vi "NIST File Header.vi"(0 "reference in":refnum<class "WaveFile.lvclass">, 5 "error in (no error)":errorcluster, 7 "Wave File Path - READ":path) -> (14 "reference out":refnum<class "WaveFile.lvclass">, 19 "error out":errorcluster)   [LabVIEW 2020, in "WaveFile.lvclass"]
uses:
  WaveFile.lvclass
panel:
  out "Header":string[](array[string])
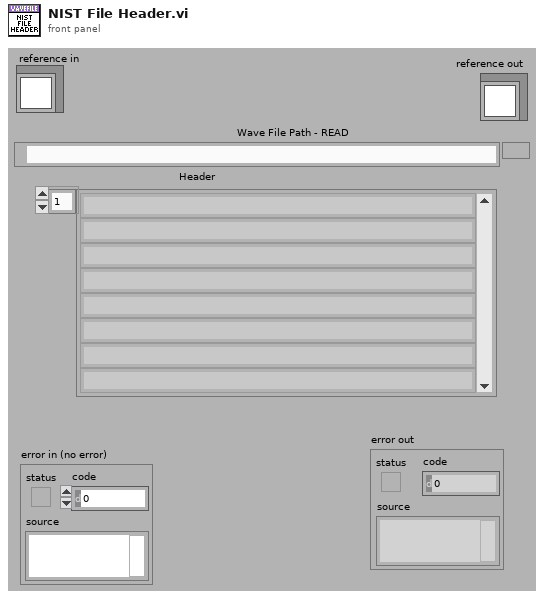
[diagram p1: front panel]
types:
  T1 = enum16{"big-endian, network order", "native, host order", "little-endian"}
  T2 = typedef "WaveFile.lvclass/ObjectAttributesRef.ctl" = refnum<data-value>
  T3 = typedef "WaveFile.lvclass/ObjectAttributes.ctl" = cluster{"Time Data":refnum<class "GSwFormDSP.lvclass">, "New Time Data Obj?":bool, "NIST File Header":T4}
  T4 = typedef "WaveFile.lvclass/NIST File Header.ctl" = cluster{"Version":string, "Header Nb Bytes":i32, "Nb Samples":i32, "Nb Bytes/sample":i32, "Nb Channels":i32, "byte order":enum16{"big-endian, network order", "native, host order", "little-endian"}, "Fs":dbl, "Valid Header?":bool}
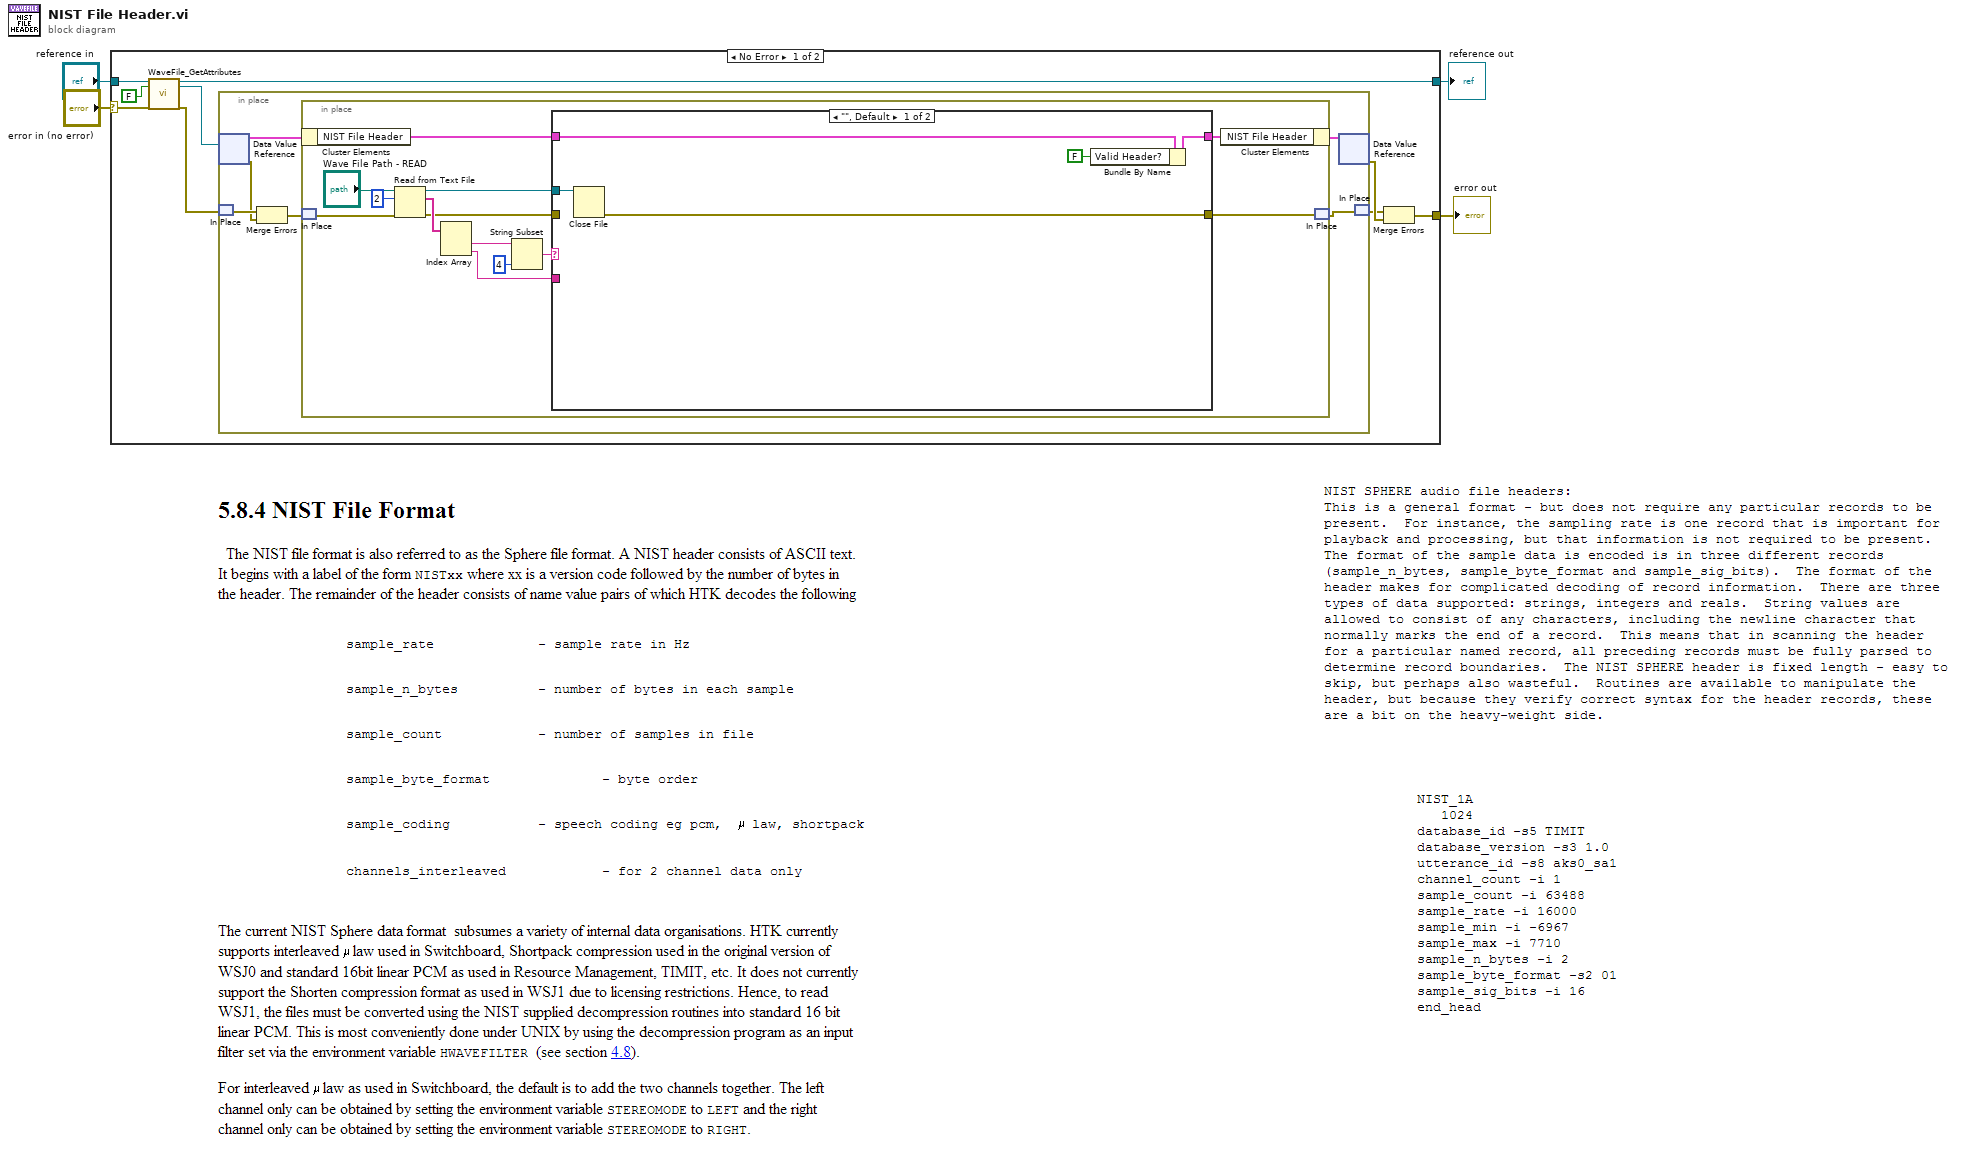
[diagram p0: block diagram]
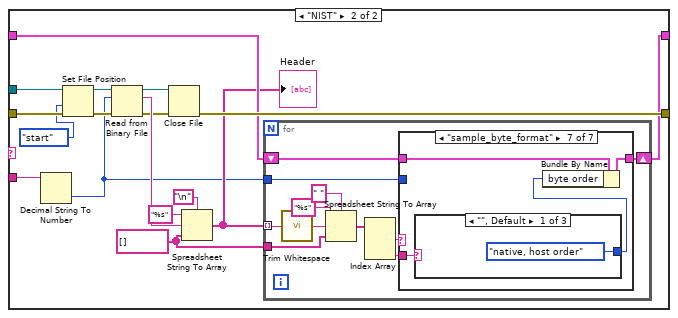
[diagram p2: hidden frame]
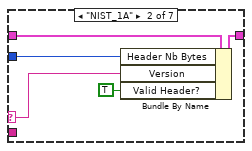
[diagram p4: hidden frame]
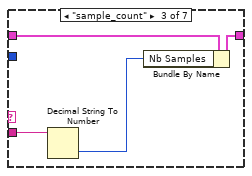
[diagram p5: hidden frame]
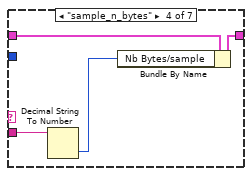
[diagram p6: hidden frame]
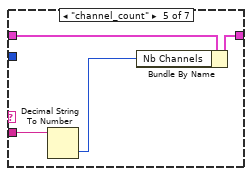
[diagram p7: hidden frame]
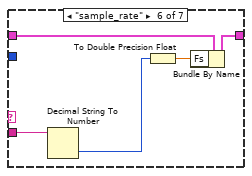
[diagram p8: hidden frame]
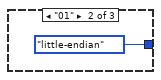
[diagram p9: hidden frame]
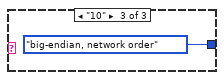
[diagram p10: hidden frame]
diagram:
  n1 = case shown="No Error" "error in (no error)" {
    selector: "error in (no error)" -> [w6 w97]
    tunnel: [w5 w97] -> w3
    tunnel: [w10 w96] -> w1
    tunnel: "reference in" -> [w12 w96]
    frame No Error {
      n2 = call "WaveFile_GetAttributes.vi"("reference in"=w12, "return data? (T)"=FALSE, "error in (no error)"=w6) -> ("reference out"=w10:refnum<class "WaveFile.lvclass">, "attributes ref"=w9:T2, "error out"=w8:errorcluster)  [unwired: 13 in, 1 out]
      n3 = in-place {
        n4 = in-place-dvr #1(w9) -> (w18:T3, w16:errorcluster)
        n5 = in-place-match #2(w8) -> (w17:errorcluster)
        n6 = Merge Errors(w17, w16) -> (w15:errorcluster)
        n7 = in-place {
          n8 = in-place-cluster #3(w18) -> ("NIST File Header"=w26:T4)
          n9 = in-place-match #4(w15) -> (w20:errorcluster)
          n10 = Read from Text File(file (use dialog)="Wave File Path - READ", count=2, error in=w20) -> (refnum out=w24:refnum<file>, text=w30:string[], error out=w23:errorcluster)  [unwired: 1 in, 1 out]
          n11 = Index Array(array=w30) -> (element #1=w29:string, element #2=w21:string)  [unwired: 2 in]
          n12 = String Subset(string=w29, length (rest)=4 ("length (rest)")) -> (substring=w27:string)  [unwired: 1 in]
          n13 = case shown="\"\", Default" w27 {
            tunnel: w26 -> [w37 w42]
            tunnel: [w35 w41] -> w25
            tunnel: w24 -> [w34 w46]
            tunnel: w23 -> [_ w47]
            tunnel: [w33 w49] -> w22
            tunnel: w21 -> [_ w48]
            frame "", Default {
              n14 = Close File(refnum=w34) -> (error out=w33:errorcluster)  [unwired: 1 in, 1 out]
              n15 = Bundle By Name(cluster=w37, "Valid Header?"=FALSE) -> (w35:T4)
            }
            frame "NIST" {
              w39 = string[] [] ("text")
              n16 = Decimal String To Number(string=w48) -> (number=w38:i32)  [unwired: 2 in, 1 out]
              n17 = Set File Position(refnum=w46, from (0:start)=enum16{"start", "end", "current"}."start", error in=w47) -> (refnum out=w45:refnum<file>, error out=w44:errorcluster)  [unwired: 1 in]
              n18 = Read from Binary File(8:w44, 10:w38, 11:w45) -> (0:w50:errorcluster, 2:w52:string, 3:w51:refnum<file>)  [unwired: 3 in, 1 out]
              n19 = Close File(refnum=w51, error in=w50) -> (error out=w49:errorcluster)  [unwired: 1 out]
              n20 = Spreadsheet String To Array(delimiter (Tab)="\n", format string="%s", spreadsheet string=w52, array type (2D Dbl)=w39) -> (array=w40:string[])
              "Header" <- w40
              n21 = for {
                shift-right: [w58] -> w41
                shift-left: w42 -> [w57]
                tunnel: w40 -> [w65] mode=indexing
                tunnel: w39 -> [w60]
                tunnel: w38 -> [w55]
                n22 = call <vilib>:"Trim Whitespace.vi"("string"=w65) -> ("trimmed string"=w64:string)  [unwired: 1 in]
                n23 = Spreadsheet String To Array(delimiter (Tab)=" ", format string="%s", spreadsheet string=w64, array type (2D Dbl)=w60) -> (array=w61:string[])
                n24 = Index Array(array=w61) -> (element #1=w59:string, element #3=w56:string)  [unwired: 3 in, 1 out]
                n25 = case shown="\"sample_byte_format\"" w59 {
                  selector: w59 -> [_ w69 _ _ _ _ _]
                  tunnel: [w66 w70 w74 w78 w82 w87 w91] -> w58
                  tunnel: w57 -> [w66 w71 w75 w79 w83 w88 w92]
                  tunnel: w56 -> [_ _ w73 w77 w81 w86 w90]
                  tunnel: w55 -> [_ w67 _ _ _ _ _]
                  frame "", Default {
                  }
                  frame "NIST_1A" {
                    n26 = Bundle By Name(cluster=w71, "Header Nb Bytes"=w67, "Version"=w69, "Valid Header?"=TRUE) -> (w70:T4)
                  }
                  frame "sample_count" {
                    n27 = Decimal String To Number(string=w73) -> (number=w72:i32)  [unwired: 2 in, 1 out]
                    n28 = Bundle By Name(cluster=w75, "Nb Samples"=w72) -> (w74:T4)
                  }
                  frame "sample_n_bytes" {
                    n29 = Decimal String To Number(string=w77) -> (number=w76:i32)  [unwired: 2 in, 1 out]
                    n30 = Bundle By Name(cluster=w79, "Nb Bytes/sample"=w76) -> (w78:T4)
                  }
                  frame "channel_count" {
                    n31 = Decimal String To Number(string=w81) -> (number=w80:i32)  [unwired: 2 in, 1 out]
                    n32 = Bundle By Name(cluster=w83, "Nb Channels"=w80) -> (w82:T4)
                  }
                  frame "sample_rate" {
                    n33 = Decimal String To Number(string=w86) -> (number=w85:i32)  [unwired: 2 in, 1 out]
                    n34 = To Double Precision Float(number=w85) -> (double precision float=w84:dbl)
                    n35 = Bundle By Name(cluster=w88, "Fs"=w84) -> (w87:T4)
                  }
                  frame "sample_byte_format" {
                    n36 = case shown="\"\", Default" w90 {
                      tunnel: [T1."native, host order" ("byte order") T1."little-endian" ("byte order") T1."big-endian, network order" ("byte order")] -> w89
                      frame "", Default {
                      }
                      frame "01" {
                      }
                      frame "10" {
                      }
                    }
                    n37 = Bundle By Name(cluster=w92, "byte order"=w89) -> (w91:T4)
                  }
                }
              }
            }
          }
          n38 = in-place-cluster #3("NIST File Header"=w25) -> (w19:T3)
          n39 = in-place-match #4(w22) -> (w14:errorcluster)
        }
        n40 = in-place-dvr #1(w19) -> (w13:errorcluster)  [unwired: 1 out]
        n41 = in-place-match #2(w14) -> (w7:errorcluster)
      }
      n42 = Merge Errors(w7, w13) -> (w5:errorcluster)
    }
    frame Error {
    }
  }
  "error out" <- w3
  "reference out" <- w1
